vi "Date Time (SubVI).vi"() -> (0 "Date & Time":string)   [LabVIEW 2015]
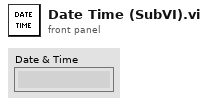
[diagram p1: front panel]
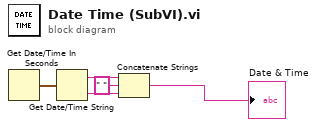
[diagram p0: block diagram]
diagram:
  n1 = Get Date/Time In Seconds() -> (seconds since 1Jan1904=w1:timestamp)
  n2 = Get Date/Time String(seconds (now)=w1) -> (date string=w2:string, time string=w3:string)  [unwired: 2 in]
  n3 = Concatenate Strings(w2, " " ("string"), w3) -> (→"Date & Time":string)
